vi "Add Labeled Points To Series.vi"(8 "error in (no error)":errorcluster, 9 "Data":cluster{"X":string, "Y":dbl}[](array[cluster])=[{"X"="", "Y"=0.25}, {"X"="", "Y"=0.75}, {"X"="", "Y"=1.95}, {"X"="", "Y"=1.6}, {"X"="", "Y"=1.6}, {"X"="", "Y"=2.5}, {"X"="", "Y"=1.8}, {"X"="", "Y"=1.26}], 11 ".NET MSChart Series":refnum<k24>) -> (0 "error out":errorcluster, 3 ".NET MSChart Series (dup)":refnum<k24>)   [LabVIEW 2014, in "XMSChart.xctl"]
uses:
  XMSChart.xctl
  System.Windows.Forms.DataVisualization
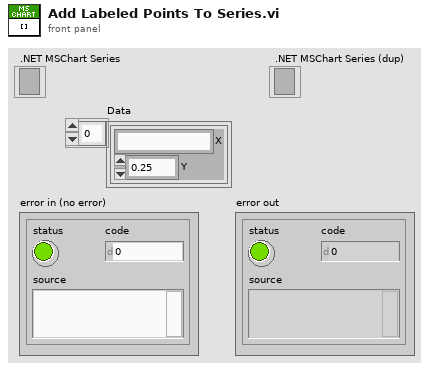
[diagram p1: front panel]
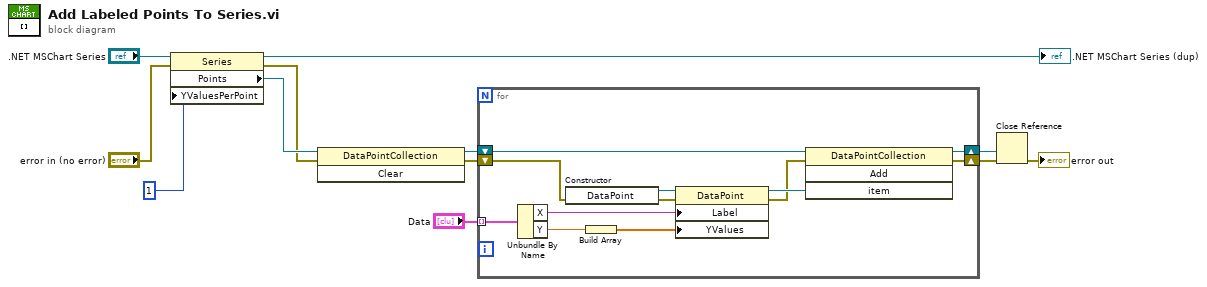
[diagram p0: block diagram]
diagram:
  n1 = property on="Property Node" class="Series"(reference=".NET MSChart Series", error in="error in (no error)", "YValuesPerPoint"=1) -> (reference out=→".NET MSChart Series (dup)":refnum<k24>, error out=w2:errorcluster, "Points"=w9:refnum<k24>)
  n2 = invoke on="Invoke Node" class="DataPointCollection" method="Clear"(reference=w9, error in=w2) -> (reference out=w3:refnum<k24>, error out=w1:errorcluster)  [unwired: 1 in, 1 out]
  n3 = for {
    tunnel: "Data" -> [w21] mode=indexing
    shift-right: [w23] -> w7
    shift-left: w3 -> [w24]
    shift-right: [w22] -> w6
    shift-left: w1 -> [w14]
    n4 = Unbundle By Name(w21) -> ("X"=w16:string, "Y"=w18:dbl)
    n5 = constructor class="DataPoint"(error in=w14) -> (reference out=w20:refnum<k24>, error out=w15:errorcluster)  [unwired: 2 in, 1 out]
    n6 = Build Array(w18) -> (w17:dbl[])
    n7 = property class="DataPoint"(reference=w20, error in=w15, "Label"=w16, "YValues"=w17) -> (reference out=w19:refnum<k24>, error out=w13:errorcluster)
    n8 = invoke class="DataPointCollection" method="Add"(reference=w24, error in=w13, "item"=w19) -> (reference out=w23:refnum<k24>, error out=w22:errorcluster)  [unwired: 1 in, 2 out]
  }
  n9 = Close Reference(reference=w7, error in (no error)=w6) -> (error out=→"error out":errorcluster)
